vi "usrednianie.vi"(3 "Wartości":dbl[](array[numeric]), 4 "AkcjaUsredniania":T2=enum."DodajWartość", 5 "Wybór Komory":T1) -> (0 "Czy kolejka pełna?":bool, 1 "Przysp. uśrednione":i32)   [LabVIEW 2014]
uses:
  akcelerometrVIs/czytajI2CVIs/usrednijVIs/AkcjaUsredniania.ctl
  parametryKomorVIs/WyborKomory.ctl
  usrednianieVIs/ParametryUsredniania.ctl
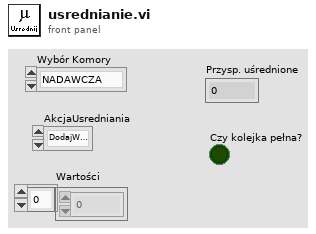
[diagram p1: front panel]
types:
  T1 = typedef "WyborKomory.ctl" = enum16{"NADAWCZA", "ODBIORCZA"}
  T2 = typedef "AkcjaUsredniania.ctl" = enum16{"Init", "DodajWartość", "WypełnijKolejkę", "Czyść"}
  T3 = typedef "ParametryUsredniania.ctl" = cluster{"Suma":dbl, "Kąty odczytane":dbl[]}
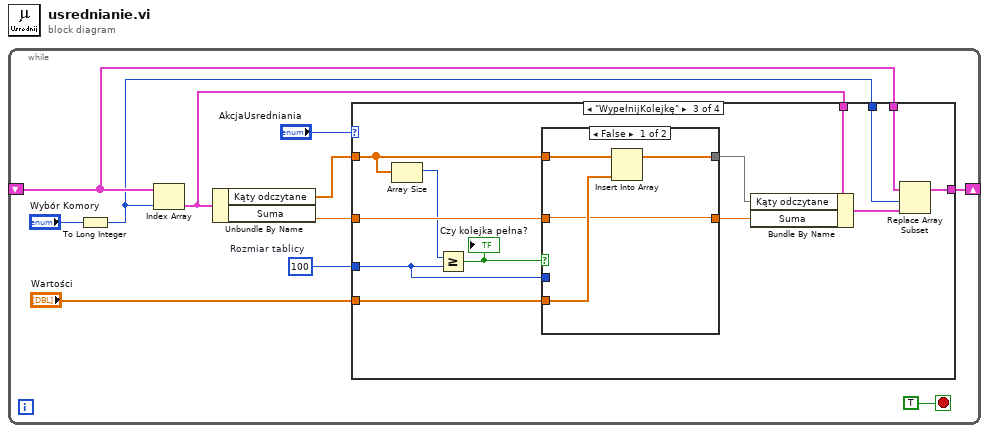
[diagram p0: block diagram]
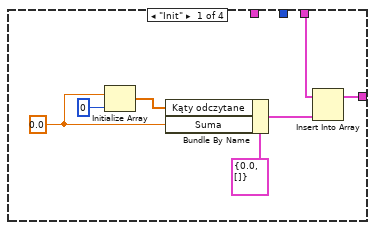
[diagram p2: hidden frame]
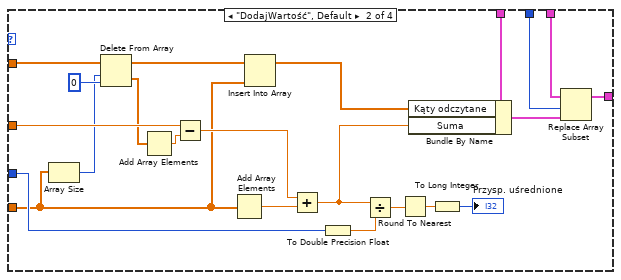
[diagram p3: hidden frame]
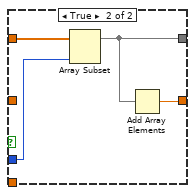
[diagram p4: hidden frame]
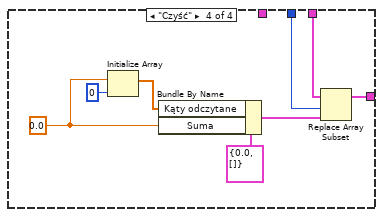
[diagram p5: hidden frame]
diagram:
  n1 = while {
    shift-right: [w10] -> _
    shift-left: _ -> [w4]
    stop <- TRUE stop-if-true
    w9 = 100  # Rozmiar tablicy
    n2 = To Long Integer(number="Wybór Komory") -> (32bit integer=w3:i32)
    n3 = Index Array(array=w4, index=w3) -> (element=w2:T3)
    n4 = Unbundle By Name(w2) -> ("Kąty odczytane"=w7:dbl[], "Suma"=w6:dbl)
    n5 = case shown="\"WypełnijKolejkę\"" "AkcjaUsredniania" {
      tunnel: w7 -> [_ w34 w50 _]
      tunnel: "Wartości" -> [_ w22 w51 _]
      tunnel: w6 -> [_ w39 w52 _]
      tunnel: [w14 w27 w45 w62] -> w10
      tunnel: w9 -> [_ w26 w41 _]
      tunnel: w4 -> [w15 w28 w44 w67]
      tunnel: w3 -> [_ w29 w43 w64]
      tunnel: w2 -> [_ w24 w42 _]
      frame "Init" {
        w16 = 0.0 ("Wartość")
        n6 = Initialize Array(w16, 0 ("dimension size")) -> (w17:dbl[])
        n7 = Bundle By Name(cluster=T3 {"Suma"=0.0, "Kąty odczytane"=[]} ("Parametry uśredniania"), "Kąty odczytane"=w17, "Suma"=w16) -> (w12:T3)
        n8 = Insert Into Array(array=w15, new element=w12) -> (w14:T3[])  [unwired: 1 in]
      }
      frame "DodajWartość", Default {
        n9 = Array Size(array=w22) -> (size(s)=w21:i32)
        n10 = Delete From Array(array=w34, length=w21, index=0) -> (deleted portion=w20:dbl[], array with subset deleted=w33:dbl[])
        n11 = Add Array Elements(numeric array=w20) -> (sum=w19:dbl)
        n12 = Subtract(x=w39, y=w19) -> (x-y=w38:dbl)
        n13 = Add Array Elements(numeric array=w22) -> (sum=w23:dbl)
        n14 = Insert Into Array(array=w33, new element=w22) -> (w31:dbl[])  [unwired: 1 in]
        n15 = Add(x=w38, y=w23) -> (x+y=w30:dbl)
        n16 = To Double Precision Float(number=w26) -> (double precision float=w40:dbl)
        n17 = Divide(x=w30, y=w40) -> (x/y=w37:dbl)
        n18 = Round To Nearest(number=w37) -> (nearest integer value=w36:dbl)
        n19 = Bundle By Name(cluster=w24, "Kąty odczytane"=w31, "Suma"=w30) -> (w32:T3)
        n20 = To Long Integer(number=w36) -> (32bit integer=→"Przysp. uśrednione":i32)
        n21 = Replace Array Subset(array=w28, new element=w32, index=w29) -> (w27:T3[])
      }
      frame "WypełnijKolejkę" {
        n22 = Array Size(array=w50) -> (size(s)=w49:i32)
        n23 = Greater Or Equal?(x=w49, y=w41) -> (x >= y?=w53:bool)
        "Czy kolejka pełna?" <- w53
        n24 = case shown="False" w53 {
          tunnel: w52 -> [w54 _]
          tunnel: w51 -> [w55 _]
          tunnel: [w54 w59] -> w47
          tunnel: w50 -> [w57 w61]
          tunnel: [w56 w58] -> w48
          tunnel: w41 -> [_ w60]
          frame False {
            n25 = Insert Into Array(array=w57, new element=w55) -> (w56:dbl[])  [unwired: 1 in]
          }
          frame True {
            n26 = Array Subset(array=w61, length=w60) -> (w58:dbl[])  [unwired: 1 in]
            n27 = Add Array Elements(numeric array=w58) -> (sum=w59:dbl)
          }
        }
        n28 = Bundle By Name(cluster=w42, "Kąty odczytane"=w48, "Suma"=w47) -> (w46:T3)
        n29 = Replace Array Subset(array=w44, new element=w46, index=w43) -> (w45:T3[])
      }
      frame "Czyść" {
        w65 = 0.0 ("Wartość")
        n30 = Initialize Array(w65, 0 ("dimension size")) -> (w66:dbl[])
        n31 = Bundle By Name(cluster=T3 {"Suma"=0.0, "Kąty odczytane"=[]} ("Parametry uśredniania"), "Kąty odczytane"=w66, "Suma"=w65) -> (w68:T3)
        n32 = Replace Array Subset(array=w67, new element=w68, index=w64) -> (w62:T3[])
      }
    }
  }
